vi "comic_crawler_tester.vi"() -> ()   [LabVIEW 2024]
uses:
  comic_crawler/status--cluster.ctl
  ComicVine_manager/status--cluster.ctl
  comic_crawler/comic_crawler.lvclass
  ComicVine_manager/ComicVine_manager.lvclass
  <vilib>/addons/_JKI Toolkits/State Machine/_JKI_lib_State_Machine.llb/Select State(s)_err__jki_lib_state_machine.vi
  003bbeb0-736b-424c-b7a2-e9a572b8fb0f.vi
  <vilib>/addons/_JKI Toolkits/State Machine/_JKI_lib_State_Machine.llb/Periodic Trigger__ogtk__JKI-SM__jki_lib_state_machine.vi
panel:
  in  "Add URL":bool
  in  "volume url":string
  out "manager status":T1
  out "size(s)":i32
  out "out of date filelist":path[](array[path])
  in  "Stop Crawler":bool
  in  "Start Crawler":bool
  out "crawler status":T2
  in  "search dirs":path[](array[path])=[path "D:/Comics/data/cv_volumes"]
  in  "Exit":bool
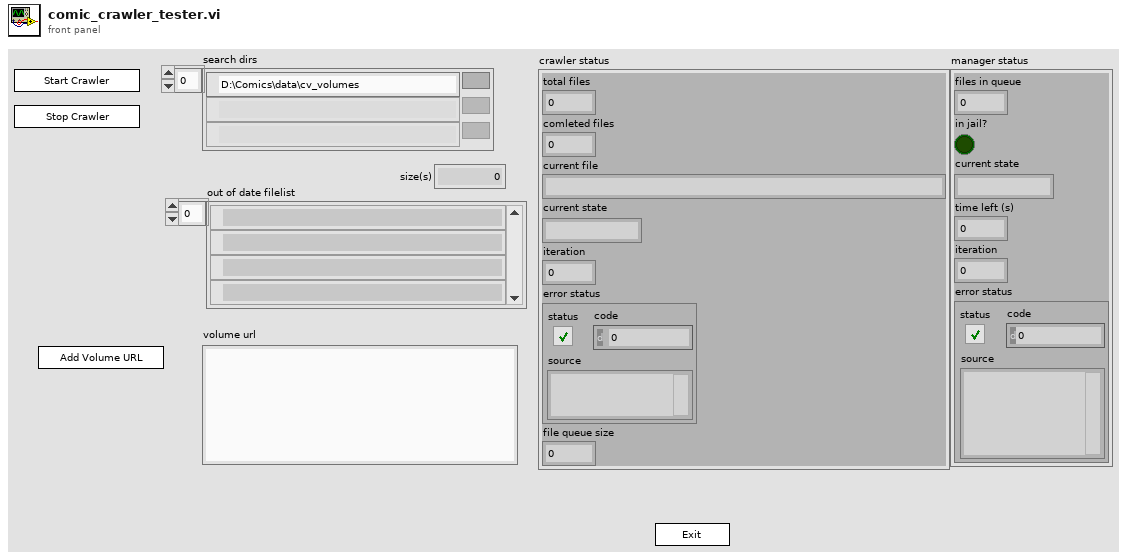
[diagram p1: front panel]
types:
  T1 = typedef "ComicVine_manager.lvclass/status--cluster.ctl" = cluster{"files in queue":i32, "in jail?":bool, "current state":string, "time left (s)":dbl, "iteration":i32, "error status":errorcluster}
  T2 = typedef "comic_crawler.lvclass/status--cluster.ctl" = cluster{"total files":i32, "comleted files":i32, "current file":string, "current state":string, "iteration":i32, "error status":errorcluster, "file queue size":i32}
  T3 = enum32{"Invalid", "Standard", "Closed", "Hidden", "Minimized", "Maximized"}
  T4 = enum32{"invalid app kind", "Development System", "Run Time System", "Student Edition", "Embedded LabVIEW", "Evaluation", "Custom"}
  T5 = cluster{"Core":cluster{"Current VI Reference":refnum<vi>, "Close Panel on Exit?":bool}, "TO":i32, "crawler":refnum<class "comic_crawler.lvclass">, "files for update":path[], "manager":refnum<class "ComicVine_manager.lvclass">, "vol_dir":path, "iss_dir":path}
  T6 = cluster{"Current VI Reference":refnum<vi>, "Close Panel on Exit?":bool}
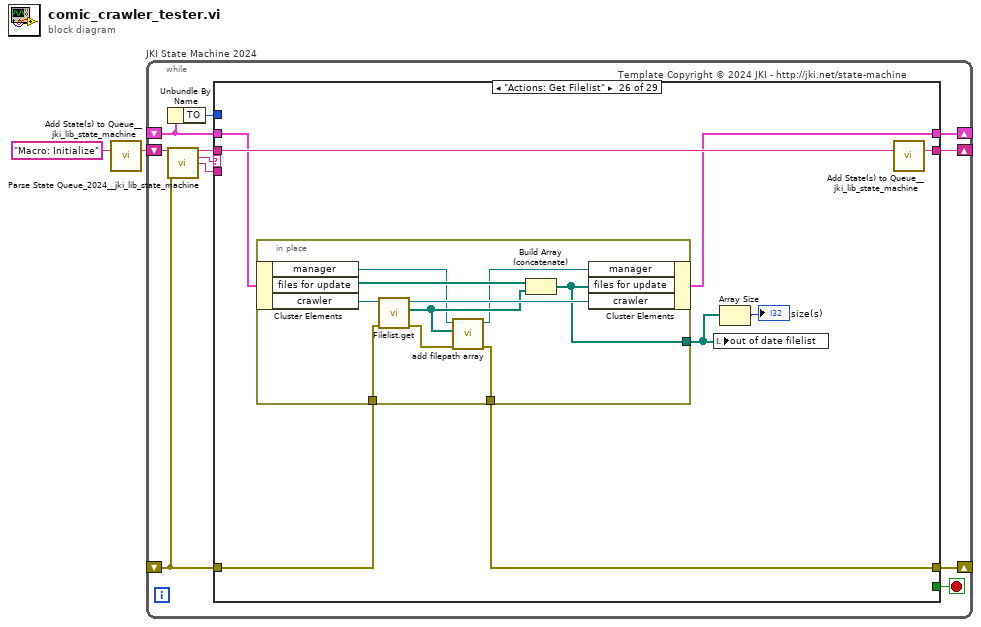
[diagram p0: block diagram]
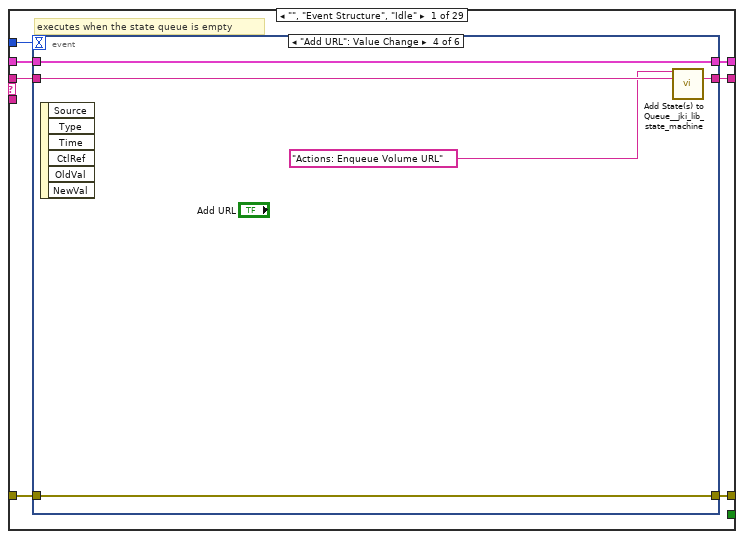
[diagram p2: hidden frame]
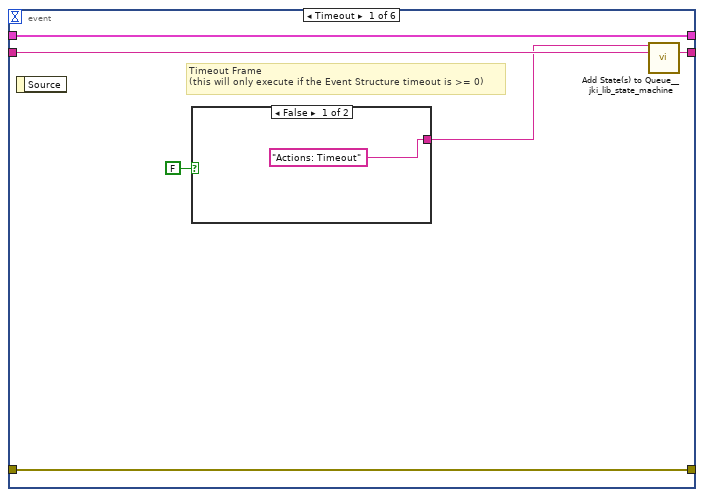
[diagram p3: hidden frame]
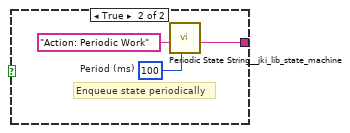
[diagram p4: hidden frame]
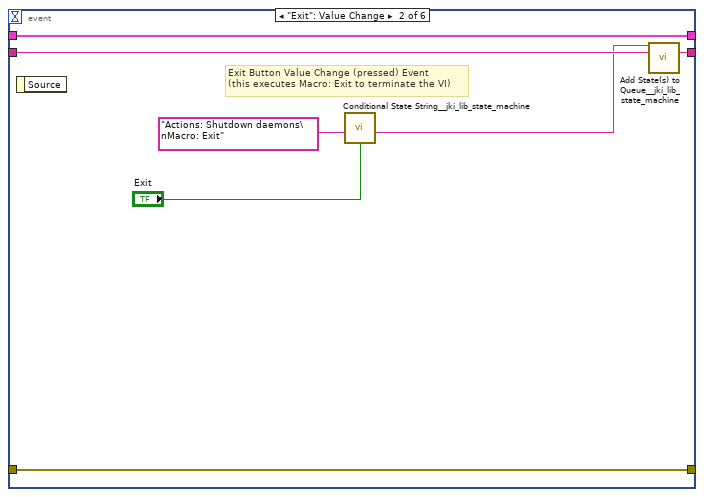
[diagram p5: hidden frame]
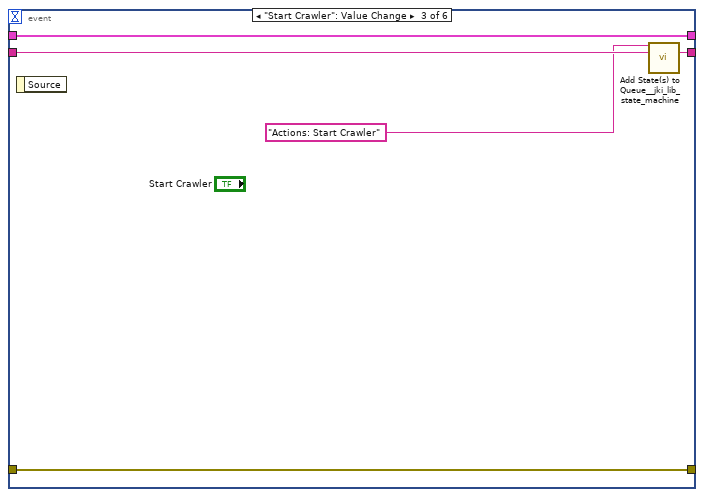
[diagram p6: hidden frame]
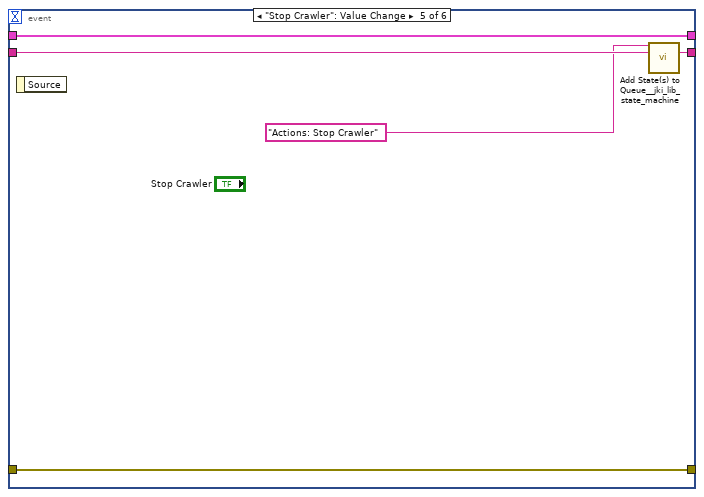
[diagram p7: hidden frame]
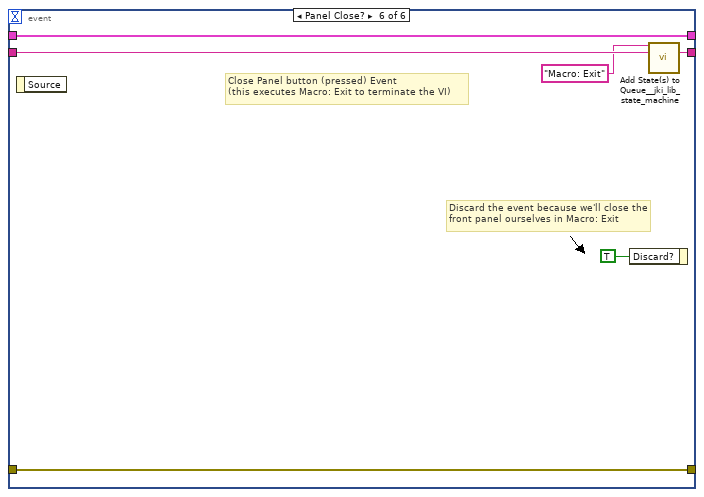
[diagram p8: hidden frame]
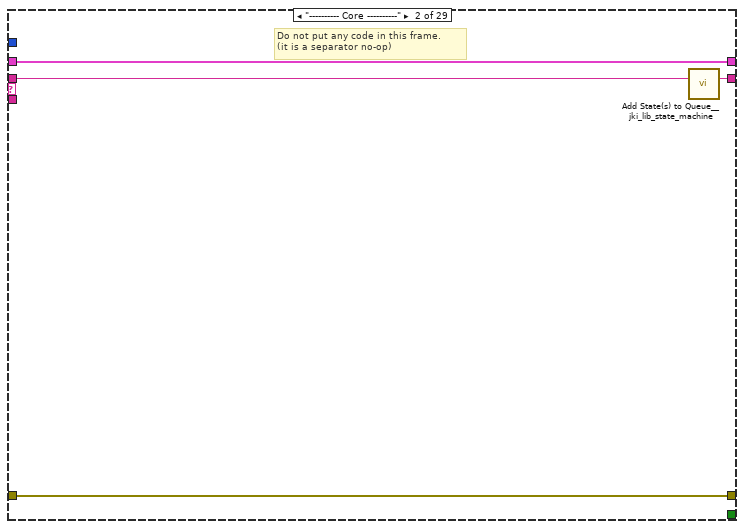
[diagram p9: hidden frame]
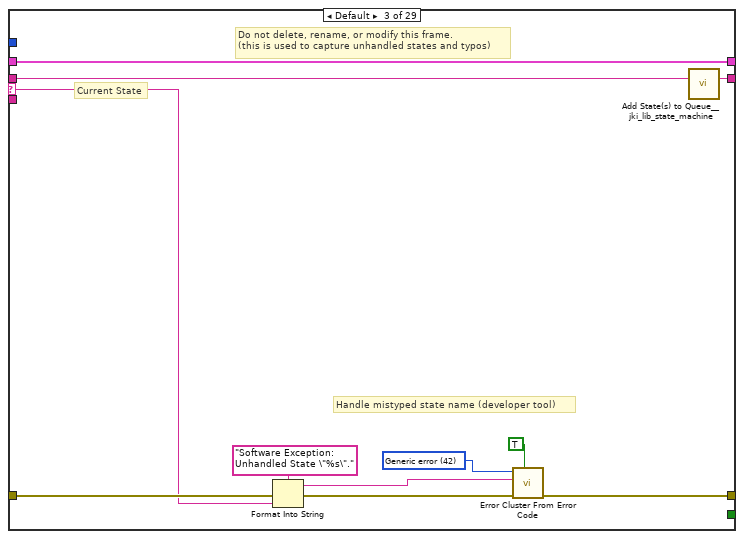
[diagram p10: hidden frame]
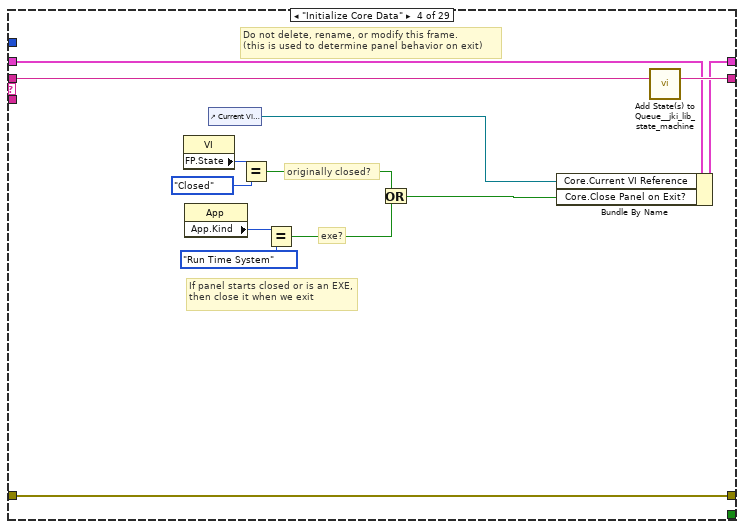
[diagram p11: hidden frame]
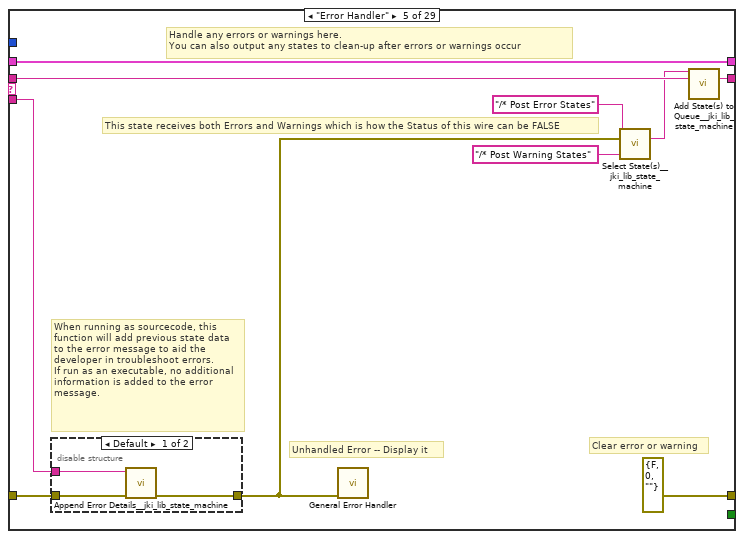
[diagram p12: hidden frame]
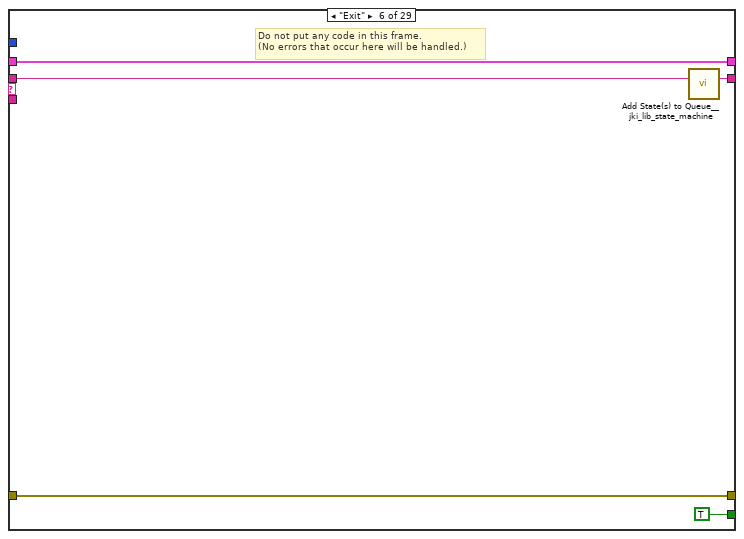
[diagram p14: hidden frame]
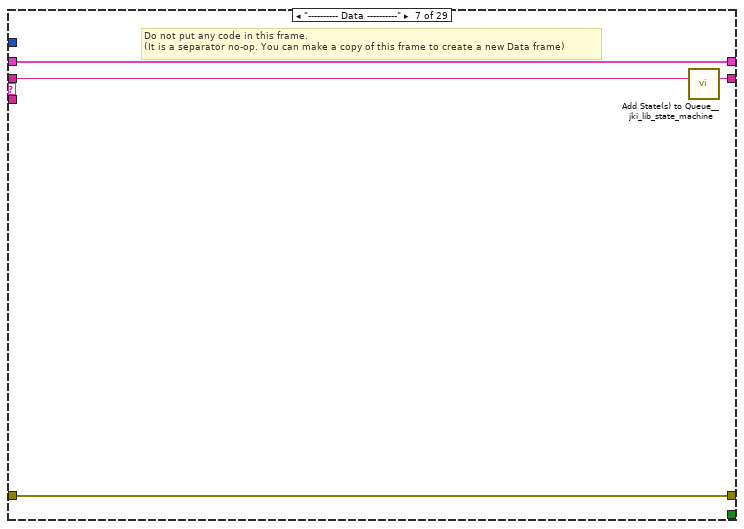
[diagram p15: hidden frame]
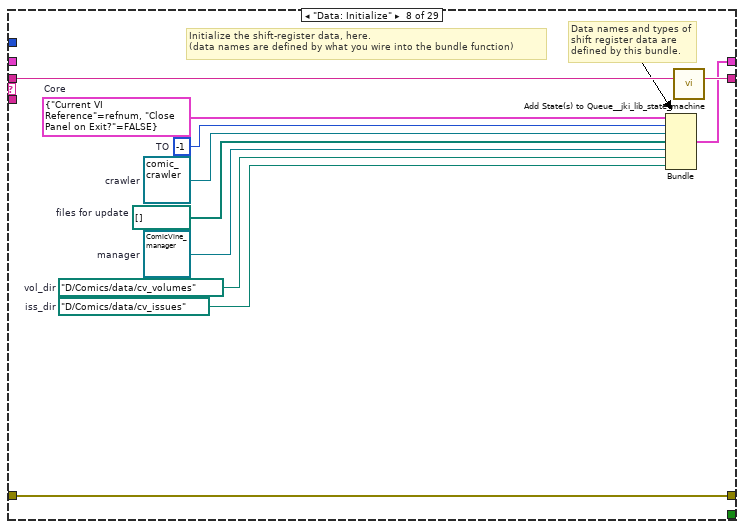
[diagram p16: hidden frame]
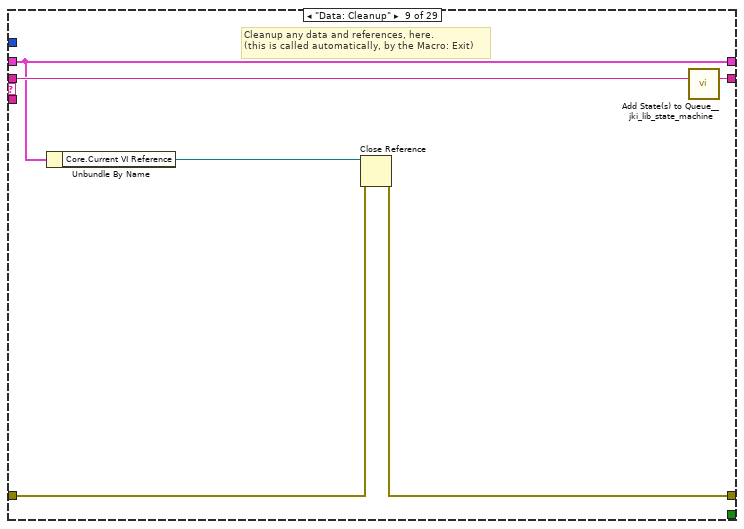
[diagram p17: hidden frame]
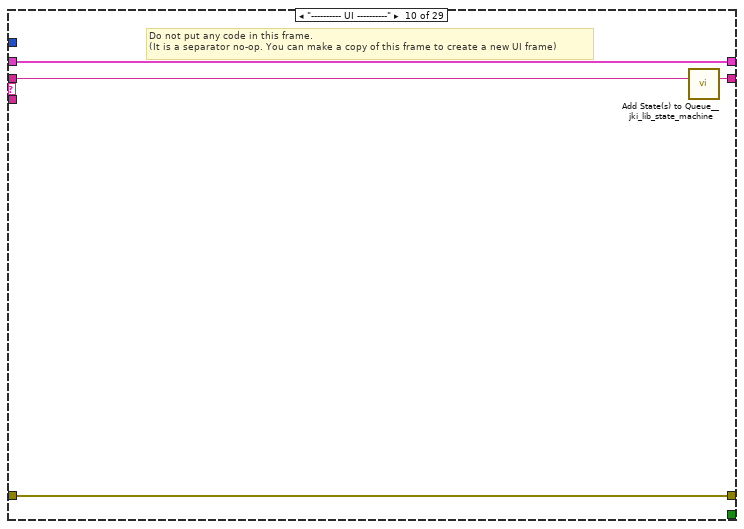
[diagram p18: hidden frame]
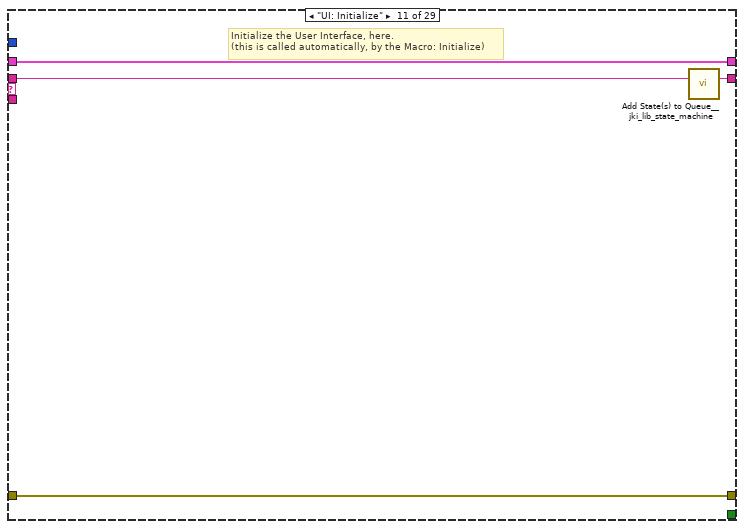
[diagram p19: hidden frame]
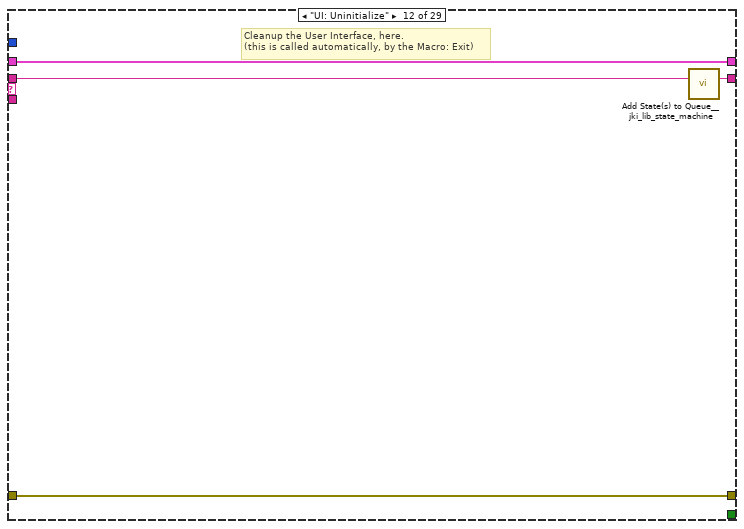
[diagram p20: hidden frame]
diagram:
  n1 = call <vilib>:"Add State(s) to Queue__jki_lib_state_machine.vi"("State(s) in (\"\")"="Macro: Initialize") -> ("States Out"=w2:string)  [unwired: 14 in]
  n2 = while "JKI State Machine 2024" {
    shift-right: [w6] -> _
    shift-left: _ -> [w4]
    shift-right: [w9] -> _
    shift-left: _ -> [w5]
    shift-right: [w8] -> _
    shift-left: w2 -> [w10]
    stop <- w7 stop-if-true
    # "Template Copyright © 2024 JKI - http://jki.net/state-machine"
    n3 = Unbundle By Name(w4) -> ("TO"=w3:i32)
    n4 = call <vilib>:"Parse State Queue_2024__jki_lib_state_machine.vi"("State Queue"=w10, "Error In (no error)"=w5) -> ("Remaining States"=w12:string, "Current State"=w13:string, "Arguments"=w11:string)  [unwired: 11 in]
    n5 = case shown="\"Actions: Get Filelist\"" w13 {
      selector: w13 -> [_ _ w63 _ _ _ _ _ _ _ _ _ _ _ _ _ _ _ _ _ _ _ _ _ _ _ _ _ _]
      tunnel: w12 -> [w20 w62 w67 w86 w96 w105 w109 w120 w126 w130 w134 w138 w144 w155 w224 w229 w238 w242 w249 w260 w269 w278 w285 w297 w310 w324 w340 w353 w365]
      tunnel: w11 -> [_ _ _ _ w91 _ _ _ _ _ _ _ w139 w149 _ _ _ _ _ _ _ _ _ _ _ _ _ _ _]
      tunnel: w4 -> [w18 w59 w65 w79 w93 w103 w106 _ w121 w127 w132 w136 w142 w151 w221 w226 w236 w239 w247 w257 w266 w272 w283 w295 w308 w322 w338 w350 w363]
      tunnel: [w17 w60 w69 w83 errorcluster {"status"=FALSE, "code"=0, "source"=""} ("error out") w102 w107 w117 w122 w128 w131 w135 w140 w152 w222 w227 w233 w240 w246 w258 w263 w274 w280 w292 w305 w317 w335 w346 w360] -> w9
      tunnel: w5 -> [w14 w60 w68 w83 w92 w102 w107 w117 w123 w128 w131 w135 w141 w153 w222 w227 w233 w240 w245 w258 w267 w275 w281 w293 w306 w320 w336 w349 w361]
      tunnel: [w19 w61 w66 w85 w95 w104 w108 w119 w125 w129 w133 w137 w143 w154 w223 w228 w237 w241 w248 w259 w268 w277 w284 w296 w309 w323 w339 w352 w364] -> w8
      tunnel: [_ _ _ _ _ TRUE _ _ _ _ _ _ _ _ _ _ _ _ _ _ _ _ _ _ _ _ _ _ _] -> w7
      tunnel: [w16 w59 w65 w84 w93 w103 w106 w118 w121 w127 w132 w136 w142 w151 w221 w226 w236 w239 w243 w257 w265 w276 w282 w294 w307 w321 w337 w350 w362] -> w6
      tunnel: w3 -> [w15 _ _ _ _ _ _ _ _ _ _ _ _ _ _ _ _ _ _ _ _ _ _ _ _ _ _ _ _]
      frame "", "Event Structure", "Idle" {
        # "executes when the state queue is empty"
        n6 = event shown="[3] \"Add URL\": Value Change" {
          selector: _ -> [_ _ _ _ _ _]
          dyn-events: _ -> [_ _ _ _ _ _]
          timeout: w15 -> [_ _ _ _ _ _]
          tunnel: w20 -> [w26 w37 w42 w47 w52 w58]
          tunnel: [w25 w36 w41 w46 w51 w57] -> w19
          tunnel: w18 -> [w23 w34 w39 w44 w49 w55]
          tunnel: [w24 w35 w40 w45 w50 w56] -> w17
          tunnel: w14 -> [w24 w35 w40 w45 w50 w56]
          tunnel: [w23 w34 w39 w44 w49 w55] -> w16
          event Timeout {
            # "Timeout Frame\n(this will only execute if the Event Structure timeout is >= 0)"
            n7 = event-data() -> ()  [unwired: 1 in, 1 out]
            n8 = case shown="False" FALSE {
              tunnel: ["Actions: Timeout" ("State Out") w30] -> w22
              frame False {
              }
              frame True {
                w28 = u32 100  # Period (ms)
                # "Enqueue state periodically"
                n9 = call <vilib>:"Periodic State String__jki_lib_state_machine.vi"("Period (ms)"=w28, "State"="Action: Periodic Work") -> ("State Out"=w30:string)  [unwired: 9 in]
              }
            }
            n10 = call <vilib>:"Add State(s) to Queue__jki_lib_state_machine.vi"("State(s) in Front (\"\")"=w22, "State(s) in (\"\")"=w26) -> ("States Out"=w25:string)  [unwired: 13 in]
          }
          event "Exit": Value Change {
            # "Exit Button Value Change (pressed) Event\n(this executes Macro: Exit to terminate the VI)"
            n11 = event-data() -> ()  [unwired: 1 in, 1 out]
            n12 = call <vilib>:"Conditional State String__jki_lib_state_machine.vi"("Do State(s)?"="Exit", "State"="Actions: Shutdown daemons\nMacro: Exit") -> ("State Out"=w31:string)  [unwired: 7 in]
            n13 = call <vilib>:"Add State(s) to Queue__jki_lib_state_machine.vi"("State(s) in Front (\"\")"=w31, "State(s) in (\"\")"=w37) -> ("States Out"=w36:string)  [unwired: 13 in]
          }
          event "Start Crawler": Value Change {
            n14 = event-data() -> ()  [unwired: 1 in, 1 out]
            n15 = call <vilib>:"Add State(s) to Queue__jki_lib_state_machine.vi"("State(s) in Front (\"\")"="Actions: Start Crawler", "State(s) in (\"\")"=w42) -> ("States Out"=w41:string)  [unwired: 13 in]
          }
          event "Add URL": Value Change {
            n16 = event-data() -> ()  [unwired: 1 in, 6 out]
            n17 = call <vilib>:"Add State(s) to Queue__jki_lib_state_machine.vi"("State(s) in Front (\"\")"="Actions: Enqueue Volume URL", "State(s) in (\"\")"=w47) -> ("States Out"=w46:string)  [unwired: 13 in]
          }
          event "Stop Crawler": Value Change {
            n18 = event-data() -> ()  [unwired: 1 in, 1 out]
            n19 = call <vilib>:"Add State(s) to Queue__jki_lib_state_machine.vi"("State(s) in Front (\"\")"="Actions: Stop Crawler", "State(s) in (\"\")"=w52) -> ("States Out"=w51:string)  [unwired: 13 in]
          }
          event Panel Close? {
            # "Discard the event because we'll close the front panel ourselves in Macro: Exit"
            # "Close Panel button (pressed) Event\n(this executes Macro: Exit to terminate the VI)"
            n20 = event-data() -> ()  [unwired: 1 in, 1 out]
            n21 = event-data("Discard?"=TRUE) -> ()  [unwired: 1 in, 1 out]
            n22 = call <vilib>:"Add State(s) to Queue__jki_lib_state_machine.vi"("State(s) in Front (\"\")"="Macro: Exit", "State(s) in (\"\")"=w58) -> ("States Out"=w57:string)  [unwired: 13 in]
          }
        }
      }
      frame "---------- Core ----------" {
        # "Do not put any code in this frame.\n(it is a separator no-op)"
        n23 = call <vilib>:"Add State(s) to Queue__jki_lib_state_machine.vi"("State(s) in (\"\")"=w62) -> ("States Out"=w61:string)  [unwired: 14 in]
      }
      frame Default {
        w72 = 42 items=["No error", "Argument error", "Memory is full", "Out of zone", "End of file", "File already open", "Generic file I/O error", "File not found", "File permission error", "Disk is full", "Duplicate path", "Too many files open", "System feature not enabled", "Resource file not found", "Cannot add resource", "Resource not found", "Image not found", "Image memory error", "Pen does not exist", "Config type invalid", "Config token not found", "Config parse error", "Config memory error", "Bad external code format", "Bad external code offset", "External code not present", "Null window", "Destroy window error", "Null menu", "Print aborted", "Bad print record", "Print driver error", "Windows error during printing", "Memory error during printing", "Print dialog error", "Generic print error", "Invalid device refnum", "Device not found", "Device parameter error", "Device unit error", "Cannot open device", "Device call aborted", "Generic error", "Cancelled by user", "Object ID too low", "Object ID too high", "Object not in heap", "Unknown heap", "Unknown object (invalid DefProc)", "Unknown object (DefProc not in table)", "Message out of range", "Invalid (null) method", "Unknown message", "Manager call not supported", "Bad address", "Network operation in progress", "Network operation timed out", "Connection is busy", "Network attribute not supported", "Network error", "Address in use", "System out of memory", "Connection aborted", "Connection refused", "Not connected", "Already connected", "Connection closed", "Initialization error (interapplication manager)", "Bad occurrence", "Wait on unbound occurrence handler", "Occurrence queue overflow", "Datalog type conflict", "Unused", "Unrecognized type (interapplication manager)", "Memory corrupt", "Failed to make temporary DLL", "Old CIN version", "Drag socket not found", "Failed to load drop-object", "Failed to register OLE object", "Failed to release OLE object", "Format specifier type mismatch", "Unknown format specifier", "Too few format specifiers", "Too many format specifiers", "Scan failed", "Newer CIN version", "Error converting to variant", "Runtime menu error", "Password tampered", "Variant attribute not found", "Incompatible variant data type", "Event data is not available", "Event Store is not present", "Occurrence is not found", "Event Queue is not created", "Event info is not available", "Refnum passed is NULL", "Error retrieving Class GUID", "Error retrieving CoClass GUID", "Error retrieving TypeLib GUID.", "Bad built application magic bytes.", "Specific driver is different from the specific driver associated with the Logical Name.", "There is no session opened to the class driver.", "Max Error", "MAX - Error with config objects", "MAX - Error loading configuration", "MAX - Group not supported"]
        # "Current State"
        # "Do not delete, rename, or modify this frame.\n(this is used to capture unhandled states and typos)"
        # "Handle mistyped state name (developer tool)"
        n24 = Format Into String(format string="Software Exception: Unhandled State \"%s\"." ("message"), error in=w68, w63) -> (resulting string=w71:string, error out=w70:errorcluster)  [unwired: 1 in]
        n25 = call <vilib>:"Error Cluster From Error Code.vi"("show call chain? (False)"=TRUE, "error in (no error)"=w70, "error message (\"\")"=w71, "error code (0)"=w72) -> ("error out"=w69:errorcluster)  [unwired: 5 in]
        n26 = call <vilib>:"Add State(s) to Queue__jki_lib_state_machine.vi"("State(s) in (\"\")"=w67) -> ("States Out"=w66:string)  [unwired: 14 in]
      }
      frame "Initialize Core Data" {
        # "Do not delete, rename, or modify this frame.\n(this is used to determine panel behavior on exit)"
        # "originally closed?"
        # "exe?"
        # "If panel starts closed or is an EXE, then close it when we exit"
        n27 = property class="VI"() -> ("FP.State"=w76:T3)  [unwired: 2 in, 2 out]
        n28 = property class="App"() -> ("App.Kind"=w82:T4)  [unwired: 2 in, 2 out]
        n29 = control-ref of="Current VI Reference"() -> (w77:refnum<vi>)
        n30 = Equal?(x=w76, y=T3."Closed" ("Front Panel Window:State")) -> (x = y?=w74:bool)
        n31 = Equal?(x=w82, y=T4."Run Time System" ("Application:Kind")) -> (x = y?=w80:bool)
        n32 = Or(x=w74, y=w80) -> (x .or. y?=w78:bool)
        n33 = Bundle By Name(cluster=w79, "Core.Current VI Reference"=w77, "Core.Close Panel on Exit?"=w78) -> (w84:T5)
        n34 = call <vilib>:"Add State(s) to Queue__jki_lib_state_machine.vi"("State(s) in (\"\")"=w86) -> ("States Out"=w85:string)  [unwired: 14 in]
      }
      frame "Error Handler" {
        # "When running as sourcecode, this function will add previous state data to the error message to aid the developer in troubleshoot errors.\nIf run as an executable, no additional information is added to the error message."
        # "This state receives both Errors and Warnings which is how the Status of this wire can be FALSE"
        # "Unhandled Error -- Display it"
        # "Handle any errors or warnings here.\nYou can also output any states to clean-up after errors or warnings occur"
        # "Clear error or warning"
        n35 = disable-structure shown="Default" {
          disable-tunnel: w92 -> [w99 w100]
          disable-tunnel: w91 -> [w98 _]
          disable-tunnel: [w97 w100] -> w90
          frame condition #0 (active) {
            n36 = call <vilib>:"Append Error Details__jki_lib_state_machine.vi"("error in (no error)"=w99, "Previous State and Argument(s)"=w98) -> ("error out"=w97:errorcluster)  [unwired: 9 in]
          }
          frame condition #1 {
          }
        }
        n37 = call <vilib>:"General Error Handler.vi"("error in (no error)"=w90) -> ()  [unwired: 10 in, 5 out]
        n38 = call-poly <vilib>:"Select State(s)__jki_lib_state_machine.vi"("State(s) if True (\"\")"="/* Post Error States", "Select"=w90, "State(s) if False (\"\")"="/* Post Warning States") -> ("States Out"=w88:string)  [unwired: 12 in]
        n39 = call <vilib>:"Add State(s) to Queue__jki_lib_state_machine.vi"("State(s) in Front (\"\")"=w88, "State(s) in (\"\")"=w96) -> ("States Out"=w95:string)  [unwired: 13 in]
      }
      frame "Exit" {
        # "Do not put any code in this frame.\n(No errors that occur here will be handled.)"
        n40 = call <vilib>:"Add State(s) to Queue__jki_lib_state_machine.vi"("State(s) in (\"\")"=w105) -> ("States Out"=w104:string)  [unwired: 14 in]
      }
      frame "---------- Data ----------" {
        # "Do not put any code in this frame.\n(It is a separator no-op. You can make a copy of this frame to create a new Data frame)"
        n41 = call <vilib>:"Add State(s) to Queue__jki_lib_state_machine.vi"("State(s) in (\"\")"=w109) -> ("States Out"=w108:string)  [unwired: 14 in]
      }
      frame "Data: Initialize" {
        w110 = path "D:/Comics/data/cv_issues"  # iss_dir
        w111 = path "D:/Comics/data/cv_volumes"  # vol_dir
        w112 = refnum<class "ComicVine_manager.lvclass"> refnum  # manager
        w113 = path[] []  # files for update
        w114 = refnum<class "comic_crawler.lvclass"> refnum  # crawler
        w115 = -1  # TO
        w116 = T6 {"Current VI Reference"=refnum, "Close Panel on Exit?"=FALSE}  # Core
        # "Data names and types of shift register data are defined by this bundle."
        # "Initialize the shift-register data, here.\n(data names are defined by what you wire into the bundle function)"
        n42 = Bundle("Core"=w116, "TO"=w115, "crawler"=w114, "files for update"=w113, "manager"=w112, "vol_dir"=w111, "iss_dir"=w110) -> (w118:T5)  [unwired: 1 in]
        n43 = call <vilib>:"Add State(s) to Queue__jki_lib_state_machine.vi"("State(s) in (\"\")"=w120) -> ("States Out"=w119:string)  [unwired: 14 in]
      }
      frame "Data: Cleanup" {
        # "Cleanup any data and references, here.\n(this is called automatically, by the Macro: Exit)"
        n44 = Unbundle By Name(w121) -> ("Core.Current VI Reference"=w124:refnum<vi>)
        n45 = Close Reference(reference=w124, error in (no error)=w123) -> (error out=w122:errorcluster)
        n46 = call <vilib>:"Add State(s) to Queue__jki_lib_state_machine.vi"("State(s) in (\"\")"=w126) -> ("States Out"=w125:string)  [unwired: 14 in]
      }
      frame "---------- UI ----------" {
        # "Do not put any code in this frame.\n(It is a separator no-op. You can make a copy of this frame to create a new UI frame)"
        n47 = call <vilib>:"Add State(s) to Queue__jki_lib_state_machine.vi"("State(s) in (\"\")"=w130) -> ("States Out"=w129:string)  [unwired: 14 in]
      }
      frame "UI: Initialize" {
        # "Initialize the User Interface, here.\n(this is called automatically, by the Macro: Initialize)"
        n48 = call <vilib>:"Add State(s) to Queue__jki_lib_state_machine.vi"("State(s) in (\"\")"=w134) -> ("States Out"=w133:string)  [unwired: 14 in]
      }
      frame "UI: Uninitialize" {
        # "Cleanup the User Interface, here.\n(this is called automatically, by the Macro: Exit)"
        n49 = call <vilib>:"Add State(s) to Queue__jki_lib_state_machine.vi"("State(s) in (\"\")"=w138) -> ("States Out"=w137:string)  [unwired: 14 in]
      }
      frame "UI: Cursor Set" {
        # "Argument"
        # "Set and Unset Cursor Busy.\n(Usage: \"UI: Cursor Set >> Busy|Idle\")"
        n50 = case shown="\"Idle\", Default" w139 {
          tunnel: w141 -> [w146 w148]
          tunnel: [w145 w147] -> w140
          frame "Idle", Default {
            n51 = call <vilib>:"Unset Busy.vi"("error in (no error)"=w146) -> ("error out"=w145:errorcluster)  [unwired: 10 in]
          }
          frame "Busy" {
            n52 = call <vilib>:"Set Busy.vi"("error in (no error)"=w148) -> ("error out"=w147:errorcluster)  [unwired: 9 in, 1 out]
          }
        }
        n53 = call <vilib>:"Add State(s) to Queue__jki_lib_state_machine.vi"("State(s) in (\"\")"=w144) -> ("States Out"=w143:string)  [unwired: 14 in]
      }
      frame "UI: Front Panel State" {
        # "Argument"
        # "Set Front Panel Open or Closed\n(Usage: \"UI: Front Panel State >> Open|Close\")"
        n54 = Unbundle By Name(w151) -> ("Core.Current VI Reference"=w150:refnum<vi>)
        n55 = case shown="\"Minimize\", \"Minimized\"" w149 {
          tunnel: w153 -> [w161 w176 w187 w200 w213]
          tunnel: [w163 w177 w189 w202 w215] -> w152
          tunnel: w150 -> [w162 w174 w188 w201 w214]
          frame "Open", "Standard", Default {
            w156 = T3."Standard" ("State")
            n56 = property class="VI"(reference=w162, error in=w161) -> (reference out=w159:refnum<vi>, error out=w160:errorcluster, "FP.State"=w158:T3)
            n57 = Not Equal?(x=w158, y=w156) -> (x != y?=w157:bool)
            n58 = case shown="True" w157 {
              tunnel: [w167 w169] -> w163
              tunnel: w160 -> [w166 w169]
              tunnel: w159 -> [w165 _]
              tunnel: w156 -> [w164 _]
              frame True {
                n59 = invoke class="VI" method="FP.Open"(reference=w165, error in=w166, "Activate"=TRUE, "State"=w164) -> (error out=w167:errorcluster)  [unwired: 1 in, 4 out]
              }
              frame False {
              }
            }
          }
          frame "Close", "Closed" {
            n60 = property class="VI"(reference=w174, error in=w176) -> (reference out=w173:refnum<vi>, error out=w175:errorcluster, "FP.State"=w171:T3)
            n61 = Not Equal?(x=w171, y=T3."Closed" ("Front Panel Window:State")) -> (x != y?=w170:bool)
            n62 = case shown="True" w170 {
              tunnel: [w178 w181] -> w177
              tunnel: w175 -> [w178 w180]
              tunnel: w173 -> [_ w179]
              frame False {
              }
              frame True {
                n63 = invoke class="VI" method="FP.Close"(reference=w179, error in=w180) -> (error out=w181:errorcluster)  [unwired: 1 in, 2 out]
              }
            }
          }
          frame "Hidden", "Hide" {
            w182 = T3."Hidden" ("State")
            n64 = property class="VI"(reference=w188, error in=w187) -> (reference out=w185:refnum<vi>, error out=w186:errorcluster, "FP.State"=w184:T3)
            n65 = Not Equal?(x=w184, y=w182) -> (x != y?=w183:bool)
            n66 = case shown="True" w183 {
              tunnel: [w193 w194] -> w189
              tunnel: w186 -> [w192 w194]
              tunnel: w185 -> [w191 _]
              tunnel: w182 -> [w190 _]
              frame True {
                n67 = invoke class="VI" method="FP.Open"(reference=w191, error in=w192, "State"=w190) -> (error out=w193:errorcluster)  [unwired: 2 in, 4 out]
              }
              frame False {
              }
            }
          }
          frame "Minimize", "Minimized" {
            w195 = T3."Minimized" ("State")
            n68 = property class="VI"(reference=w201, error in=w200) -> (reference out=w198:refnum<vi>, error out=w199:errorcluster, "FP.State"=w197:T3)
            n69 = Not Equal?(x=w197, y=w195) -> (x != y?=w196:bool)
            n70 = case shown="True" w196 {
              tunnel: [w206 w207] -> w202
              tunnel: w199 -> [w205 w207]
              tunnel: w198 -> [w204 _]
              tunnel: w195 -> [w203 _]
              frame True {
                n71 = invoke class="VI" method="FP.Open"(reference=w204, error in=w205, "State"=w203) -> (error out=w206:errorcluster)  [unwired: 2 in, 4 out]
              }
              frame False {
              }
            }
          }
          frame "Maximize", "Maximized" {
            w208 = T3."Maximized" ("State")
            n72 = property class="VI"(reference=w214, error in=w213) -> (reference out=w211:refnum<vi>, error out=w212:errorcluster, "FP.State"=w210:T3)
            n73 = Not Equal?(x=w210, y=w208) -> (x != y?=w209:bool)
            n74 = case shown="True" w209 {
              tunnel: [w219 w220] -> w215
              tunnel: w212 -> [w218 w220]
              tunnel: w211 -> [w217 _]
              tunnel: w208 -> [w216 _]
              frame True {
                n75 = invoke class="VI" method="FP.Open"(reference=w217, error in=w218, "State"=w216) -> (error out=w219:errorcluster)  [unwired: 2 in, 4 out]
              }
              frame False {
              }
            }
          }
        }
        n76 = call <vilib>:"Add State(s) to Queue__jki_lib_state_machine.vi"("State(s) in (\"\")"=w155) -> ("States Out"=w154:string)  [unwired: 14 in]
      }
      frame "---------- Macro ----------" {
        # "Do not put any code in this frame.\n(It is a separator no-op. You can make a copy of this frame to create a new Macro frame)"
        n77 = call <vilib>:"Add State(s) to Queue__jki_lib_state_machine.vi"("State(s) in (\"\")"=w224) -> ("States Out"=w223:string)  [unwired: 14 in]
      }
      frame "Macro: Initialize" {
        w225 = "Data: Initialize\nInitialize Core Data\nUI: Initialize\nUI: Front Panel State >> Open\nActions: Create Crawler\nActions: Launch Crawler\nActions: Create Manager\nActions: Launch Manager"  # Data: Initialize Initialize Core Data UI: Initialize UI: Front Panel State >> Open Actions: Create Crawler Actions: Launch Crawler Actions: Create Manager Actions: Launch Manager
        # "Initialization Macro\n(This is called once, when the VI starts)"
        n78 = call <vilib>:"Add State(s) to Queue__jki_lib_state_machine.vi"("State(s) in Front (\"\")"=w225, "State(s) in (\"\")"=w229) -> ("States Out"=w228:string)  [unwired: 13 in]
      }
      frame "Macro: Exit" {
        # "Exit Macro\n(This is called once, when the VI exits)"
        n79 = Unbundle By Name(w236) -> ("Core.Close Panel on Exit?"=w231:bool)
        n80 = call <vilib>:"Conditional State String__jki_lib_state_machine.vi"("Do State(s)?"=w231, "State"="UI: Front Panel State >> Close") -> ("State Out"=w230:string)  [unwired: 7 in]
        n81 = call <vilib>:"Add State(s) to Queue__jki_lib_state_machine.vi"("State(s) in (\"\")"=w230, "State(s) at Back (\"\")"="UI: Uninitialize\nData: Cleanup\nExit") -> ("States Out"=w234:string)  [unwired: 13 in]
        n82 = call <vilib>:"Add State(s) to Queue__jki_lib_state_machine.vi"("State(s) in Front (\"\")"=w234, "State(s) in (\"\")"=w238) -> ("States Out"=w237:string)  [unwired: 13 in]
      }
      frame "---------- Actions ----------" {
        # "Template Separator\n(You can make a copy of, or modify, this frame)"
        n83 = call <vilib>:"Add State(s) to Queue__jki_lib_state_machine.vi"("State(s) in (\"\")"=w242) -> ("States Out"=w241:string)  [unwired: 14 in]
      }
      frame "Actions: Enqueue Volume URL" {
        n84 = in-place {
          in-place-border: w245 -> [w254]
          in-place-border: [w253] -> w246
          in-place-border: "volume url" -> [w250]
          n85 = in-place-cluster #1(w247) -> ("iss_dir"=w252:path, "vol_dir"=w251:path, "manager"=w256:refnum<class "ComicVine_manager.lvclass">)
          n86 = call "add volume by URL.vi"("volume parent dir"=w251, "issue parent dir"=w252, "error in (no error)"=w254, "URL"=w250, "ComicVine_manager in"=w256) -> ("error out"=w253:errorcluster, "ComicVine_manager out"=w255:refnum<class "ComicVine_manager.lvclass">)  [unwired: 5 in]
          n87 = in-place-cluster #1("iss_dir"=w252, "vol_dir"=w251, "manager"=w255) -> (w243:T5)
        }
        n88 = call <vilib>:"Add State(s) to Queue__jki_lib_state_machine.vi"("State(s) in (\"\")"=w249) -> ("States Out"=w248:string)  [unwired: 14 in]
      }
      frame "Actions: Periodic Action" {
        n89 = call <vilib>:"Add State(s) to Queue__jki_lib_state_machine.vi"("State(s) in (\"\")"=w260) -> ("States Out"=w259:string)  [unwired: 14 in]
      }
      frame "Actions: Create Crawler" {
        n90 = call "create.vi"("error in"=w267, "delay (s)"=2.0) -> ("error out"=w263:errorcluster, "comic_crawler.lvclass"=w264:refnum<class "comic_crawler.lvclass">)  [unwired: 8 in]
        n91 = Bundle By Name(cluster=w266, "TO"=-1, "crawler"=w264) -> (w265:T5)
        n92 = call <vilib>:"Add State(s) to Queue__jki_lib_state_machine.vi"("State(s) in (\"\")"=w269) -> ("States Out"=w268:string)  [unwired: 14 in]
      }
      frame "Actions: Create Manager" {
        n93 = Unbundle By Name(w272) -> ("vol_dir"=w271:path, "iss_dir"=w270:path)
        n94 = call "create.vi"("error in (no error)"=w275, "issue directory"=w270, "volume directory"=w271) -> ("error out"=w274:errorcluster, "ComicVine_manager out"=w273:refnum<class "ComicVine_manager.lvclass">)  [unwired: 7 in]
        n95 = Bundle By Name(cluster=w272, "manager"=w273) -> (w276:T5)
        n96 = call <vilib>:"Add State(s) to Queue__jki_lib_state_machine.vi"("State(s) in (\"\")"=w278) -> ("States Out"=w277:string)  [unwired: 14 in]
      }
      frame "Actions: Launch Crawler" {
        n97 = in-place {
          in-place-border: w281 -> [w288]
          in-place-border: [w287] -> w280
          in-place-border: 100 ("Tester Timeout") -> [w286]
          n98 = in-place-cluster #2(w283) -> ("crawler"=w290:refnum<class "comic_crawler.lvclass">)  [unwired: 1 out]
          n99 = call "Launch.vi"("error in (no error)"=w288, "comic_crawler in"=w290) -> ("error out"=w287:errorcluster, "comic_crawler out"=w289:refnum<class "comic_crawler.lvclass">)  [unwired: 8 in]
          n100 = in-place-cluster #2("crawler"=w289, "TO"=w286) -> (w282:T5)
        }
        n101 = call <vilib>:"Add State(s) to Queue__jki_lib_state_machine.vi"("State(s) in (\"\")"=w285) -> ("States Out"=w284:string)  [unwired: 14 in]
      }
      frame "Actions: Launch Manager" {
        n102 = in-place {
          in-place-border: w293 -> [w299]
          in-place-border: [w298] -> w292
          in-place-border: 100 ("Tester Timeout") -> [w302]
          n103 = in-place-cluster #3(w295) -> ("manager"=w301:refnum<class "ComicVine_manager.lvclass">)  [unwired: 1 out]
          n104 = call "Launch.vi"("error in (no error)"=w299, "ComicVine_manager in"=w301) -> ("error out"=w298:errorcluster, "ComicVine_manager out"=w300:refnum<class "ComicVine_manager.lvclass">)  [unwired: 8 in]
          n105 = in-place-cluster #3("manager"=w300, "TO"=w302) -> (w294:T5)
        }
        n106 = call <vilib>:"Add State(s) to Queue__jki_lib_state_machine.vi"("State(s) in (\"\")"=w297) -> ("States Out"=w296:string)  [unwired: 14 in]
      }
      frame "Actions: Start Crawler" {
        n107 = in-place {
          in-place-border: w306 -> [w314]
          in-place-border: [w313] -> w305
          in-place-border: "search dirs" -> [w312]
          in-place-border: [w311] -> w303
          w311 = path[] [] ("files for update")
          n108 = in-place-cluster #4(w308) -> ("crawler"=w316:refnum<class "comic_crawler.lvclass">)  [unwired: 1 out]
          n109 = call "Start.vi"("error in (no error)"=w314, "search dirs"=w312, "comic_crawler in"=w316) -> ("error out"=w313:errorcluster, "comic_crawler out"=w315:refnum<class "comic_crawler.lvclass">)  [unwired: 7 in]
          n110 = in-place-cluster #4("files for update"=w311, "crawler"=w315) -> (w307:T5)
        }
        "out of date filelist" <- w303
        n111 = call <vilib>:"Add State(s) to Queue__jki_lib_state_machine.vi"("State(s) in (\"\")"=w310) -> ("States Out"=w309:string)  [unwired: 14 in]
      }
      frame "Actions: Get Filelist" {
        n112 = in-place {
          in-place-border: w320 -> [w332]
          in-place-border: [w330] -> w319
          in-place-border: [w325] -> w317
          n113 = in-place-cluster #5(w322) -> ("manager"=w327:refnum<class "ComicVine_manager.lvclass">, "files for update"=w331:path[], "crawler"=w334:refnum<class "comic_crawler.lvclass">)
          n114 = call "Filelist.get.vi"("error in (no error)"=w332, "comic_crawler in"=w334) -> ("error out"=w328:errorcluster, "out of date filelist"=w329:path[], "comic_crawler out"=w333:refnum<class "comic_crawler.lvclass">)  [unwired: 7 in]
          n115 = call "add filepath array.vi"("error in (no error)"=w328, "filepath array"=w329, "ComicVine_manager in"=w327) -> ("error out"=w325:errorcluster, "ComicVine_manager out"=w326:refnum<class "ComicVine_manager.lvclass">)  [unwired: 7 in]
          n116 = Build Array (concatenate)(w331, w329) -> (w330:path[])
          n117 = in-place-cluster #5("manager"=w326, "files for update"=w330, "crawler"=w333) -> (w321:T5)
        }
        n118 = local write "out of date filelist"(w319) -> ()
        n119 = Array Size(array=w319) -> (size(s)=→"size(s)":i32)
        n120 = call <vilib>:"Add State(s) to Queue__jki_lib_state_machine.vi"("State(s) in (\"\")"=w324) -> ("States Out"=w323:string)  [unwired: 14 in]
      }
      frame "Actions: Stop Crawler" {
        n121 = in-place {
          in-place-border: w336 -> [w342]
          in-place-border: [w341] -> w335
          n122 = in-place-cluster #6(w338) -> ("crawler"=w344:refnum<class "comic_crawler.lvclass">)
          n123 = call "Stop.vi"("error in (no error)"=w342, "comic_crawler in"=w344) -> ("error out"=w341:errorcluster, "comic_crawler out"=w343:refnum<class "comic_crawler.lvclass">)  [unwired: 8 in]
          n124 = in-place-cluster #6("crawler"=w343) -> (w337:T5)
        }
        n125 = call <vilib>:"Add State(s) to Queue__jki_lib_state_machine.vi"("State(s) in (\"\")"=w340) -> ("States Out"=w339:string)  [unwired: 14 in]
      }
      frame "Actions: Shutdown daemons" {
        n126 = Unbundle By Name(w350) -> ("manager"=w345:refnum<class "ComicVine_manager.lvclass">, "crawler"=w351:refnum<class "comic_crawler.lvclass">)
        n127 = call "destroy.vi"("comic_crawler in"=w351) -> ("error out"=w347:errorcluster)  [unwired: 10 in]
        n128 = call "destroy.vi"("ComicVine_manager in"=w345) -> ("error out"=w348:errorcluster)  [unwired: 10 in]
        n129 = Merge Errors(w349, w348, w347) -> (w346:errorcluster)
        n130 = call <vilib>:"Add State(s) to Queue__jki_lib_state_machine.vi"("State(s) in (\"\")"=w353) -> ("States Out"=w352:string)  [unwired: 14 in]
      }
      frame "Actions: Timeout" {
        n131 = in-place {
          in-place-border: [w373] -> w358
          in-place-border: w361 -> [w371]
          in-place-border: [w367] -> w360
          in-place-border: [w366] -> w354
          n132 = in-place-cluster #7(w363) -> ("manager"=w370:refnum<class "ComicVine_manager.lvclass">, "crawler"=w374:refnum<class "comic_crawler.lvclass">)
          n133 = call "Status.get.vi"("error in (no error)"=w371, "comic_crawler in"=w374) -> ("error out"=w368:errorcluster, "current status"=w373:T2, "comic_crawler out"=w372:refnum<class "comic_crawler.lvclass">)  [unwired: 7 in]
          n134 = call "Status.get.vi"("error in (no error)"=w368, "ComicVine_manager in"=w370) -> ("error out"=w367:errorcluster, "current status"=w366:T1, "ComicVine_manager out"=w369:refnum<class "ComicVine_manager.lvclass">)  [unwired: 7 in]
          n135 = in-place-cluster #7("manager"=w369, "crawler"=w372) -> (w362:T5)
        }
        "crawler status" <- w358
        "manager status" <- w354
        n136 = Unbundle By Name(w358) -> ("file queue size"=w359:i32)
        n137 = call "Is Value Changed.vim"("value"=w359) -> ("changed or first call?"=w357:bool)
        n138 = call <vilib>:"Conditional State String__jki_lib_state_machine.vi"("Do State(s)?"=w357, "State"="Actions: Get Filelist") -> ("State Out"=w356:string)  [unwired: 7 in]
        n139 = call <vilib>:"Add State(s) to Queue__jki_lib_state_machine.vi"("State(s) in Front (\"\")"=w356, "State(s) in (\"\")"=w365) -> ("States Out"=w364:string)  [unwired: 13 in]
      }
    }
  }
